vi "Set Enable.vi"(8 "error in (no error)":errorcluster, 10 "Enable":bool, 11 "Fault-Insertion_Type in":refnum<class "Fault-Injection_Type.lvclass">) -> (0 "error out":errorcluster, 3 "Fault-Insertion_Type out":refnum<class "Fault-Injection_Type.lvclass">)   [LabVIEW 2021, in "Fault-Injection_Type.lvclass"]
uses:
  Fault-Injection_Type.lvclass
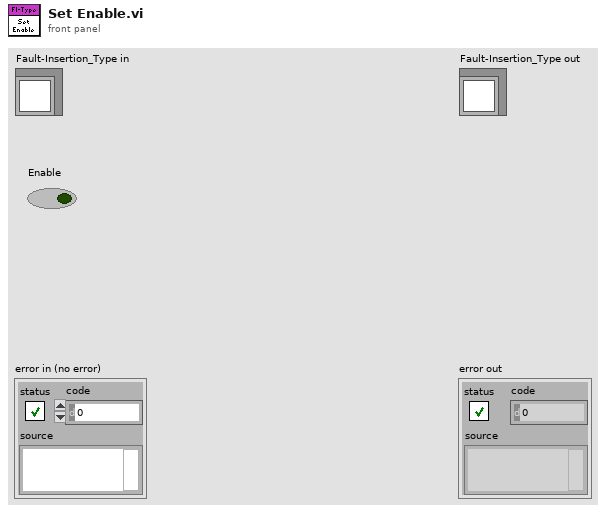
[diagram p1: front panel]
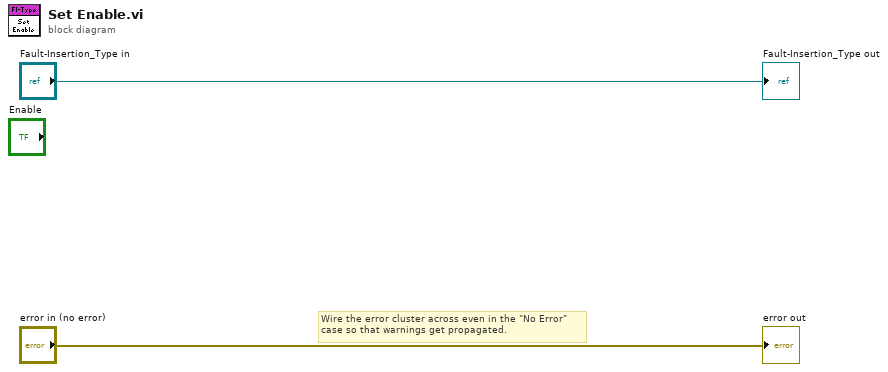
[diagram p0: block diagram]
diagram:
  # "Wire the error cluster across even in the \"No Error\"\ncase so that warnings get propagated."
  "error out" <- "error in (no error)"
  "Fault-Insertion_Type out" <- "Fault-Insertion_Type in"
